vi "test.vi"   [LabVIEW 2017]
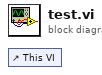
[diagram p0: block diagram]
diagram:
  n1 = control-ref of="This VI"() -> ()  [unwired: 1 out]
